vi "plot_XY.vi"(0 "reference":refnum<class "OSA.lvclass">, 1 "X-data":sgl[](array[numeric]), 2 "Y-data":sgl[](array[numeric]), 3 "autoScale X (True)":bool, 4 "autoScale Y (True)":bool, 5 "error in (no error)":errorcluster, 6 "Label X-scale":string="X label", 7 "skip":bool, 8 "Label Y-scale":string="Y label", 9 "error rangeViolation":bool, 11 "class compatible (True)":bool=TRUE, 13 "graph properties":T2) -> (14 "duplicate reference":refnum<class "OSA.lvclass">, 19 "error out":errorcluster={"status"=TRUE, "code"=5000, "source"="\nNot enough nr of data points in acqusition or plot data.\r\n[Thorlabs_FTS_LV61_plot_data_update.vi->Thorlabs_FTS_LV61_plot_update.vi->Thorlabs_FTS_LV61_plot_spectrum.vi->Thorlabs_FTS_LV61_example_asyncAcqusition.vi]"})   [LabVIEW 2010, in "OSA.lvclass"]
doc: "In the case 'class compatible' is true; the Y-data will be plotted in an intensity graph which corresponding reference has been provided/routed to the init.vi Graph Spectrum terminal, (default dataacquisition spectrum graph). \n\nOr if 'class compatible' is false; the graph properties must be provided by the 'graph properties' control. \n\nSetting class compatible to False is useful for graphs in parallell with the data aqquisition graph, (data acquisition graph reference provided to init.vi).\n\nA compatible intensity graph can be found in the tree.vi.\n\nX and Y data must be provided/routed, (as opposed to none XY plotting vis, where data is provided from the dataAcquisition buffer)."
uses:
  OSA.lvclass
  private/graph_intensity.ctl
  OSA20X_misc.lvlib
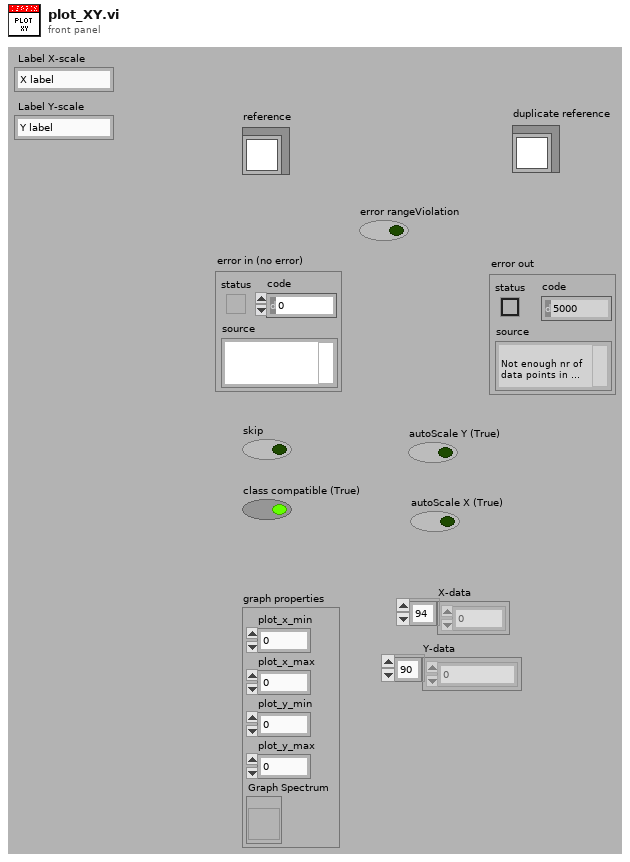
[diagram p1: front panel]
types:
  T1 = typedef "OSA.lvclass/graph_intensity.ctl" = refnum<vi>
  T2 = cluster{"plot_x_min":sgl, "plot_x_max":sgl, "plot_y_min":sgl, "plot_y_max":sgl, "Graph Spectrum":T1}
  T3 = typedef "OSA.lvclass/ObjectAttributes.ctl" = cluster{"Stop":bool, "dataType":T4, "spectrometerIdx":u16, "buffer size interferogram":i32, "interferogram":cluster{"new":bool, "plot_x_ min":sgl, "plot_x_max":sgl, "plot_y_min":sgl, "plot_y_max":sgl, "Graph Intrfrgrm":T1, "timeStamp":u32, "signal (%)":dbl, "traces":cluster{"idx":u32, "broadBand":bool, "monoChromatic":bool, "peakToPeakSignal":dbl, "peakToPeakPos":dbl}[], "traces idx last":i32, "contrast (%)":dbl}, "spectrum":cluster{"new":bool, "plot_x_min":sgl, "plot_x_max":sgl, "plot_unit_x":T5, "plot_unit_y":T6, "plot_y_min":sgl, "plot_y_max":sgl, "Graph Spectrum":T1, "timeStamp":u32, "X_VAL_OPTIONS":enum16{"MIN_MAX", "ARRAY"}, "traces":cluster{"idx":u32}[], "traces idx last":i32}, "Thorlabs_OSA_64.lvclass:queue_action.ctlqueue ref":refnum<queue>, "action":T7, "plot zoom step":dbl, "buffer semaphore":T8, "acq stopped":bool, "dataType active":T4, "temperature (degr C)":sgl, "pressure (hPa)":sgl, "rel humidity (%)":sgl, "settings":cluster{"resolution":u16, "sensitivity":u16, "Average":bool, "average nr":u32, "apodisation":T9, "acq delay (ms)":u32, "airMesure":T10, "wmtr on":bool, "intfgrm_smooth_width":u16, "intfgrm_smooth_nrOfPasses":u16, "intfgrm_smooth":T11, "phaseCorrection":T12, "zeroFill":u8, "spectr_smooth":T11, "spectr_smooth_width":u16, "spectr_smooth_nrOfPasses":u16, "resolution (/cm)":sgl, "REF wavelength, (nm)":dbl, "gain_idx":u16, "gainAuto":bool, "gain_relative":dbl, "PD sensitivity mode":T13, "PD senseMode implemented":bool, "SensorTemperature implemented":bool, "SensorPressure implemented":bool, "SensorHumidity implemented":bool, "attenuationAuto":bool, "attenuationOnOff":bool, "attenuationAvailable":bool, "offsetAvailable":bool, "offset":i32, "offset max":u16, "contrastAvailable":bool}, "peaks position":sgl[], "peaks width":sgl[], "peaks height":sgl[], "peaks max nr":u32, "peaks latest nr":i32, "peaks new":bool, "power":dbl, "power new":bool, "path":string, "wavelength (WNr)":dbl, "wavelength new":bool, "buffer size spectrum":i32, "status":string, "vi reference":refnum<vi>, "funcPointer":u64, "libraryPointer":u64, "singleAcquisition":bool, "coherenceLength (cm)":dbl, "coherenceLength new":bool, "spectrometer model":string, "spectrometer serial nr":string, "peaks thld left":sgl[], "peaks thld right":sgl[], "coherenceLength error (cm)":dbl, "ADC bits":u16, "peaks position centroid":sgl[], "peaks height centroid":sgl[], "OSA series":T14, "channel index spectrum":u16, "spectrometer rangeLow, (/cm)":dbl, "spectrometer rangeHigh, (/cm)":dbl, "channel index interferogram":u16, "virtualSource":bool, "sweep restart":bool}
  T4 = typedef "OSA.lvclass/acq_dataType.ctl" = enum16{"none", "interferogram", "spectrum"}
  T5 = typedef "OSA.lvclass/spectrum_x_unit.ctl" = enum16{"wavenr/cm", "THz", "eV", "nm_air", "nm_vac"}
  T6 = typedef "OSA.lvclass/y_unit.ctl" = enum16{"ADC counts", "dBm pwr absolute", "dBm pwr density", "mW pwr absolute", "mW pwr density"}
  T7 = typedef "OSA.lvclass/queue_action.ctl" = enum16{"none", "stop", "GUI_plotInterferogram", "GUI_plotSpectrum", "GUI_plotInterferogramRescale", "GUI_plotSpectrumRescale", "GUI_plotInterferogramReset", "GUI_plotSpectrumReset", "GUI_plotInterferogramAutoScaleY", "GUI_plotSpectrumAutoScaleY", "GUI_plotInterferogramZoomOut", "GUI_plotSpectrumZoomOut", "GUI_plotInterferogramPane", "GUI_plotSpectrumPane", "GUI_plotInterferogramZoomMouse", "GUI_plotSpectrumZoomMouse", "GUI_plotSpectrumFSRY", "GUI_plotInterferogramFSRY", "GUI_spectrumChannelType", "GUI_channel", "ENVIRONMENT temperature", "ENVIRONMENT pressure", "MODE_resolution set", "MODE_resolution get", "MODE_sensitivity set", "MODE_sensitivity get", "MODE_PDTemperature set", "MODE_PDTemperature get", "REBOOT/RESET firmware", "ACQASYNC_acquireSingleSpectrum", "ACQASYNC_continuous start", "ACQASYNC_continuous stop\n", "ACQASYNC_get last interferogram", "ACQASYNC_get last spectrum", "ACQASYNC_get last waveNr", "ACQOPT_interferogram smoothing set", "ACQOPT_interferogram smoothing get", "ACQOPT_spectrum smoothing set", "ACQOPT_spectrum smoothing get", "ACQOPT_apodisation type set", "ACQOPT_apodisation type get", "ACQOPT_phase correction type set", "ACQOPT_phase correction type get", "ACQOPT_acqIntervall_set", "ACQOPT_acqIntervall_get", "ACQOPT_average spectrum set", "ACQOPT_average spectrum get", "ACQOPT_rolling average set", "ACQOPT_rolling average get", "ACQOPT_zero fill factor set", "ACQOPT_zero fill factor get", "ACQOPT_cycle counting set", "ACQOPT_cycle counting get", "ACQOPT_air measure option set", "ACQOPT_air measure option get", "ACQOPT_gainLevel auto get", "ACQOPT_gainLevel auto set", "ACQOPT_gainLevel get", "ACQOPT_gainLevel set", "ACQOPT_offset set", "ACQOPT_attenuator_auto_set", "ACQOPT_attenuator_set", "ACQOPT_getAll", "INSTRUMENT_PROPERTY_range_WaveNr_min", "INSTRUMENT_PROPERTY_range_WaveNr_max", "INSTRUMENT_PROPERTY_reference_wavelength_cm^-1", "INSTRUMENT_PROPERTY_samplesPerRefPeriod", "INSTRUMENT_PROPERTY_resolution_waveNrPercm", "INSTRUMENT_PROPERTY_availableGainLevels", "INSTRUMENT_PROPERTY_status", "CONVERT", "ANALYSE_POWER", "ANALYSE_PEAKS", "ANALYSE_WAVELENGTH", "ANALYSE_SPECTRUM", "ANALYSE_INTERFEROGRAM", "ANALYSE_COHERENCE_LENGTH", "MATH", "MATH_power", "MATH_peaks", "FILE", "miscellaneous"}
  T8 = typedef "Semaphore RefNum" = refnum<k1>
  T9 = typedef "OSA.lvclass/apodisation.ctl" = enum16{"NONE", "NORTON_BEER_WEAK", "NORTON_BEER_MEDIUM", "NORTON_BEER_STRONG", "TRIANGULAR", "COSINE", "HANN", "HAMMING", "BLACKMANHARRIS3", "BLACKMANHARRIS4", "GAUSSIAN"}
  T10 = typedef "OSA.lvclass/airMeasure.ctl" = enum16{"TEMPERATURE", "PRESSURE"}
  T11 = typedef "OSA20X_misc.lvlib/interferogram_smoothing.ctl" = enum16{"NONE", "BINOMIAL", "SAVITSKY_GOLAY", "FOURIER", "MOVING_AVERAGE", "GAUSSIAN"}
  T12 = typedef "OSA.lvclass/phaseCorrection.ctl" = enum16{"NONE", "MERTZ", "FORMAN", "MERTZ_FILE", "FORMAN_FILE", "FUTURE COMP."}
  T13 = typedef "OSA20X_misc.lvlib/PDTemperatureMode.ctl" = enum16{"cool: better sensitivity/noise floor", "warm: extended wl range"}
  T14 = typedef "OSA.lvclass/OSA_series.ctl" = enum16{"OSA200", "OSA300", "UNKNOWN"}
  T15 = cluster{"new":bool, "plot_x_min":sgl, "plot_x_max":sgl, "plot_unit_x":T5, "plot_unit_y":T6, "plot_y_min":sgl, "plot_y_max":sgl, "Graph Spectrum":T1, "timeStamp":u32, "X_VAL_OPTIONS":enum16{"MIN_MAX", "ARRAY"}, "traces":cluster{"idx":u32}[], "traces idx last":i32}
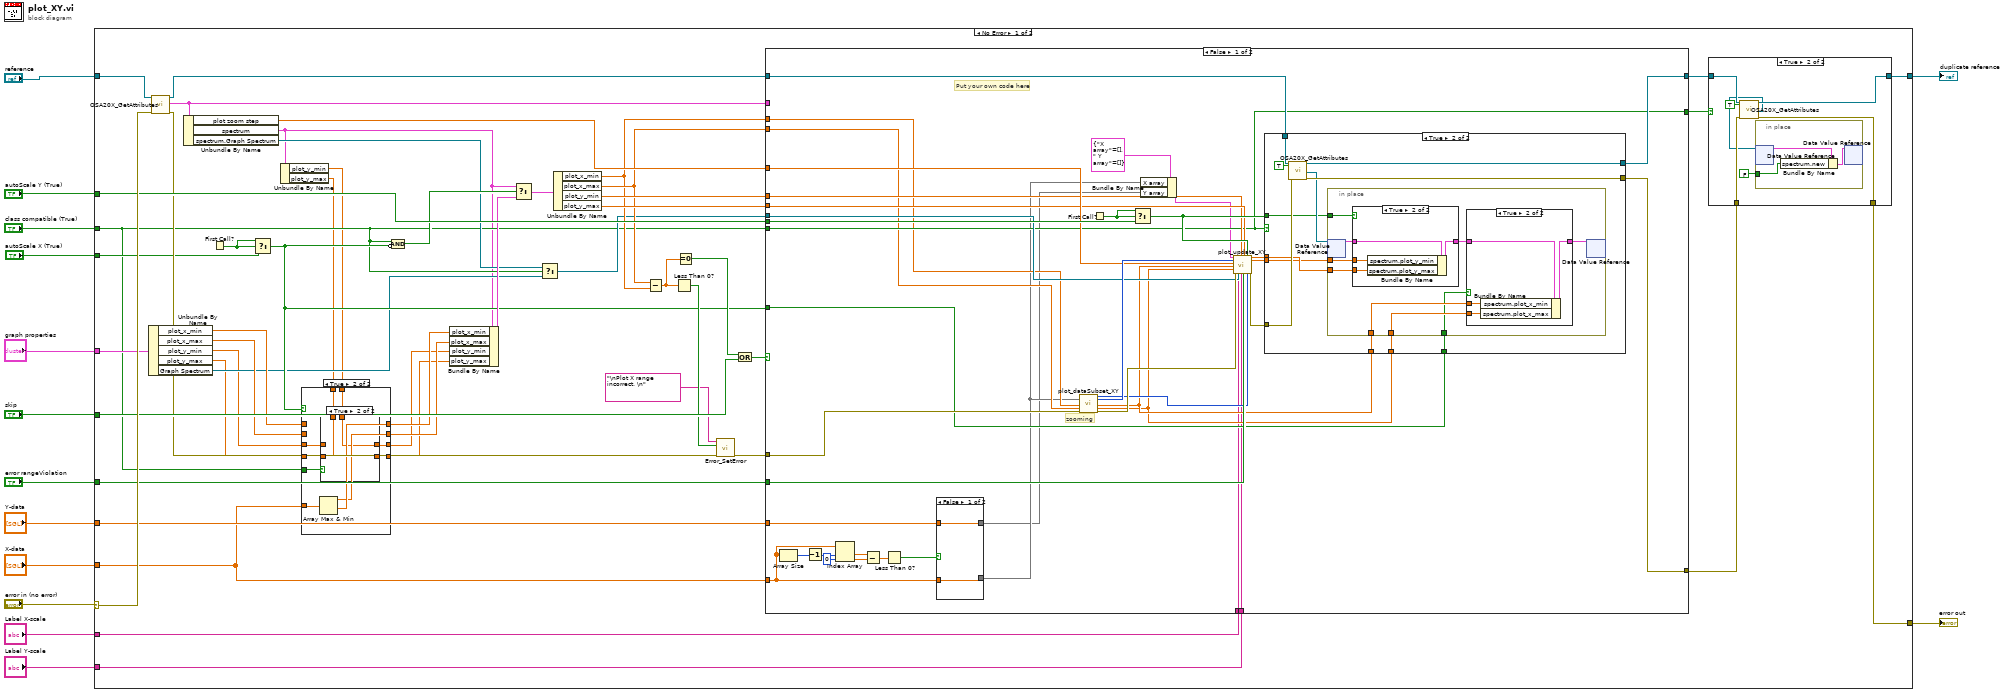
[diagram p0: block diagram]
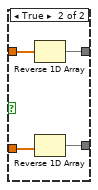
[diagram p5: hidden frame]
diagram:
  n1 = case shown="No Error" "error in (no error)" {
    selector: "error in (no error)" -> [w63 w176]
    tunnel: [w59 w176] -> w14
    tunnel: "reference" -> [w64 w177]
    tunnel: [w58 w177] -> w11
    tunnel: "error rangeViolation" -> [w62 _]
    tunnel: "autoScale Y (True)" -> [w61 _]
    tunnel: "skip" -> [w53 _]
    tunnel: "class compatible (True)" -> [w22 _]
    tunnel: "graph properties" -> [w49 _]
    tunnel: "Y-data" -> [w54 _]
    tunnel: "autoScale X (True)" -> [w34 _]
    tunnel: "X-data" -> [w25 _]
    tunnel: "Label X-scale" -> [w16 _]
    tunnel: "Label Y-scale" -> [w15 _]
    frame No Error {
      n2 = Unbundle By Name(w49) -> ("plot_x_min"=w33:sgl, "plot_x_max"=w32:sgl, "plot_y_min"=w24:sgl, "plot_y_max"=w23:sgl, "Graph Spectrum"=w27:T1)
      n3 = call "OSA20X_GetAttributes.vi"("reference in"=w64, "error in (no error)"=w63) -> ("reference out"=w56:refnum<class "OSA.lvclass">, "Data"=w50:T3, "error out"=w43:errorcluster)  [unwired: 14 in, 1 out]
      n4 = Unbundle By Name(w50) -> ("plot zoom step"=w48:dbl, "spectrum"=w21:T15, "spectrum.Graph Spectrum"=w28:T1)
      n5 = First Call?() -> (First Call?: T/F=w36:bool)
      n6 = Select(t=w36, s=w36, f=w34) -> (s? t:f=w31:bool)
      n7 = Unbundle By Name(w21) -> ("plot_y_min"=w19:sgl, "plot_y_max"=w20:sgl)
      n8 = case shown="True" w31 {
        tunnel: w33 -> [w67 _]
        tunnel: w32 -> [w68 _]
        tunnel: [w67 w77] -> w30
        tunnel: [w68 w76] -> w29
        tunnel: w25 -> [_ w78]
        tunnel: w24 -> [w66 w74]
        tunnel: w23 -> [w65 w73]
        tunnel: w22 -> [_ w75]
        tunnel: w20 -> [_ w72]
        tunnel: w19 -> [_ w71]
        tunnel: [w66 w70] -> w18
        tunnel: [w65 w69] -> w17
        frame False {
        }
        frame True {
          n9 = Array Max & Min(array=w78) -> (max value=w76:sgl, min value=w77:sgl)  [unwired: 2 out]
          n10 = case shown="True" w75 {
            tunnel: w74 -> [w80 _]
            tunnel: w73 -> [w79 _]
            tunnel: w72 -> [_ w81]
            tunnel: w71 -> [_ w82]
            tunnel: [w80 w82] -> w70
            tunnel: [w79 w81] -> w69
            frame False {
            }
            frame True {
            }
          }
        }
      }
      n11 = Compound Arithmetic op=AND(w22, invert w31) -> (w35:bool)
      n12 = Bundle By Name(cluster=w21, "plot_x_min"=w30, "plot_x_max"=w29, "plot_y_min"=w18, "plot_y_max"=w17) -> (w52:T15)
      n13 = Select(t=w21, s=w35, f=w52) -> (s? t:f=w51:T15)
      n14 = Select(t=w28, s=w22, f=w27) -> (s? t:f=w26:T1)
      n15 = Unbundle By Name(w51) -> ("plot_x_min"=w44:sgl, "plot_x_max"=w45:sgl, "plot_y_min"=w46:sgl, "plot_y_max"=w47:sgl)
      n16 = Subtract(x=w45, y=w44) -> (x-y=w39:sgl)
      n17 = Less Than 0?(x=w39) -> (x < 0?=w41:bool)
      n18 = Equal To 0?(x=w39) -> (x = 0?=w38:bool)
      n19 = call "Error_SetError.vi"("error in"=w43, "status (true)"=w41, "source(\"\")"="\nPlot X range incorrect. \n" ("source(\"\")")) -> ("error out"=w42:errorcluster)  [unwired: 4 in]
      n20 = Or(x=w38, y=w53) -> (x .or. y?=w55:bool)
      n21 = case shown="False" w55 {
        tunnel: [w133 w175] -> w57
        tunnel: [w131 w174] -> w60
        tunnel: w50 -> [_ _]
        tunnel: w62 -> [w128 _]
        tunnel: w61 -> [w126 _]
        tunnel: w56 -> [w125 w175]
        tunnel: w22 -> [w115 w173]
        tunnel: w54 -> [w96 _]
        tunnel: w48 -> [w120 _]
        tunnel: w47 -> [w119 _]
        tunnel: w46 -> [w118 _]
        tunnel: w44 -> [w113 _]
        tunnel: w45 -> [w112 _]
        tunnel: w42 -> [w117 w174]
        tunnel: w26 -> [w116 _]
        tunnel: [w115 w173] -> w37
        tunnel: w31 -> [w110 _]
        tunnel: w25 -> [w98 _]
        tunnel: w16 -> [w107 _]
        tunnel: w15 -> [w106 _]
        frame False {
          # "zooming"
          # "Put your own code here"
          n22 = Array Size(array=w98) -> (size(s)=w105:i32)
          n23 = Decrement(x=w105) -> (x-1=w104:i32)
          n24 = Index Array(array=w98, index #1=w104, index #2=0 ("index")) -> (element #1=w102:sgl, element #2=w101:sgl)
          n25 = Subtract(x=w102, y=w101) -> (x-y=w100:sgl)
          n26 = Less Than 0?(x=w100) -> (x < 0?=w99:bool)
          n27 = case shown="False" w99 {
            tunnel: w98 -> [w134 w139]
            tunnel: w96 -> [w135 w138]
            tunnel: [w135 w137] -> w95
            tunnel: [w134 w136] -> w97
            frame False {
            }
            frame True {
              n28 = Reverse 1D Array(array=w138) -> (reversed array=w137:sgl[])
              n29 = Reverse 1D Array(array=w139) -> (reversed array=w136:sgl[])
            }
          }
          n30 = call "plot_dataSubset_XY.vi"("X-data"=w97, "zoom range low"=w113, "zoom range high"=w112, "error in (no error)"=w117) -> ("idx start"=w124:i32, "length"=w129:i32, "X min actual"=w114:sgl, "X max actual"=w111:sgl, "error out"=w130:errorcluster)  [unwired: 11 in]
          n31 = First Call?() -> (First Call?: T/F=w127:bool)
          n32 = Select(t=w127, s=w127, f=w126) -> (s? t:f=w123:bool)
          n33 = Bundle By Name(cluster=cluster{"X array":sgl[], " Y array":sgl[]} {"X array"=[], " Y array"=[]} ("data"), "X array"=w97, "Y array"=w95) -> (w108:cluster{"X array":sgl[], " Y array":sgl[]})
          n34 = call "plot_update_XY.vi"("data"=w108, "data length"=w129, "x zoom factor"=w120, "X range min"=w114, "X range max"=w111, "error in (no error)"=w130, "graph ref"=w116, "X Scale.Name Label.Text"=w107, "y range min"=w118, "Y Scale.Name Label.Text"=w106, "y range max"=w119, "error rangeViolation"=w128, "autoScale Y"=w123, "data idxStart"=w124) -> ("dataVal max"=w122:sgl, "dataVal min"=w121:sgl, "error out"=w132:errorcluster)  [unwired: 3 in]
          n35 = case shown="True" w115 {
            tunnel: [w141 w153] -> w133
            tunnel: w132 -> [w140 w152]
            tunnel: [w140 w151] -> w131
            tunnel: w125 -> [w141 w150]
            tunnel: w123 -> [_ w147]
            tunnel: w122 -> [_ w146]
            tunnel: w121 -> [_ w145]
            tunnel: w114 -> [_ w144]
            tunnel: w111 -> [_ w143]
            tunnel: w110 -> [_ w142]
            frame False {
            }
            frame True {
              n36 = call "OSA20X_GetAttributes.vi"("reference in"=w150, "OnlyGetDvrReference(False)"=TRUE, "error in (no error)"=w152) -> ("reference out"=w153:refnum<class "OSA.lvclass">, "DataRef"=w148:refnum<data-value>, "error out"=w151:errorcluster)  [unwired: 13 in, 1 out]
              n37 = in-place {
                in-place-border: w147 -> [w162]
                in-place-border: w146 -> [w160]
                in-place-border: w145 -> [w159]
                in-place-border: w144 -> [w156]
                in-place-border: w143 -> [w155]
                in-place-border: w142 -> [w154]
                n38 = in-place-dvr #1(w148) -> (w161:T3)  [unwired: 1 out]
                n39 = case shown="True" w162 {
                  tunnel: w161 -> [w168 w172]
                  tunnel: [w168 w171] -> w158
                  tunnel: w160 -> [_ w170]
                  tunnel: w159 -> [_ w169]
                  frame False {
                  }
                  frame True {
                    n40 = Bundle By Name(cluster=w172, "spectrum.plot_y_min"=w169, "spectrum.plot_y_max"=w170) -> (w171:T3)
                  }
                }
                n41 = case shown="True" w154 {
                  tunnel: w158 -> [w163 w167]
                  tunnel: [w163 w166] -> w157
                  tunnel: w156 -> [_ w165]
                  tunnel: w155 -> [_ w164]
                  frame False {
                  }
                  frame True {
                    n42 = Bundle By Name(cluster=w167, "spectrum.plot_x_min"=w165, "spectrum.plot_x_max"=w164) -> (w166:T3)
                  }
                }
                n43 = in-place-dvr #1(w157) -> ()  [unwired: 2 out]
              }
            }
          }
        }
        frame True {
        }
      }
      n44 = case shown="True" w37 {
        tunnel: w60 -> [w84 w91]
        tunnel: [w84 w90] -> w59
        tunnel: [w83 w89] -> w58
        tunnel: w57 -> [w83 w88]
        frame False {
        }
        frame True {
          n45 = call "OSA20X_GetAttributes.vi"("reference in"=w88, "OnlyGetDvrReference(False)"=TRUE, "error in (no error)"=w91) -> ("reference out"=w89:refnum<class "OSA.lvclass">, "DataRef"=w86:refnum<data-value>, "error out"=w90:errorcluster)  [unwired: 13 in, 1 out]
          n46 = in-place {
            in-place-border: FALSE ("dataNewIntrfrgrm") -> [w93]
            n47 = in-place-dvr #2(w86) -> (w94:T3)  [unwired: 1 out]
            n48 = Bundle By Name(cluster=w94, "spectrum.new"=w93) -> (w92:T3)
            n49 = in-place-dvr #2(w92) -> ()  [unwired: 2 out]
          }
        }
      }
    }
    frame Error {
      # "Error"
    }
  }
  "error out" <- w14
  "duplicate reference" <- w11
